vi "SnapShoot.vi"(8 "error in (no error)":errorcluster, 11 "CameraTestingProxy in":refnum<class "CameraTestingProxyAPI.lvclass">) -> (0 "error out":errorcluster, 2 "SnapData":T1, 3 "CameraTestingProxy out":refnum<class "CameraTestingProxyAPI.lvclass">)   [LabVIEW 2020, in "CameraTestingProxy.lvlib" / "CameraTestingProxyAPI.lvclass"]
uses:
  CameraTestingProxyAPI.lvclass
  ICameraTestingProxy/TypeDef/SnapData.ctl
  ICameraTestingProxy/TypeDef/Resolution.ctl
  CameraTestingProxyAPI.lvclass/CameraTestingProxyAPI.ctl
  81c5d912-67c1-434d-ab51-26c85ecb9ac1.vi
  ICameraTestingProxy/TypeDef/ICameraTestingProxy_typedef.lvlib
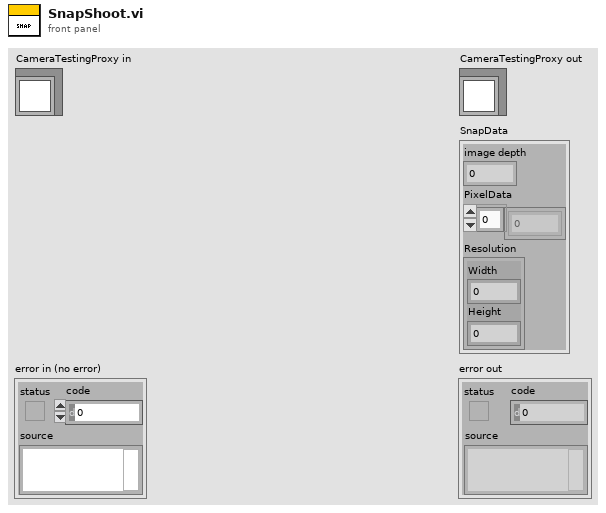
[diagram p1: front panel]
types:
  T1 = typedef "ICameraTestingProxy_typedef.lvlib/SnapData.ctl" = cluster{"image depth":i32, "PixelData":u8[], "Resolution":T2}
  T2 = typedef "ICameraTestingProxy_typedef.lvlib/Resolution.ctl" = cluster{"Width":i16, "Height":i16}
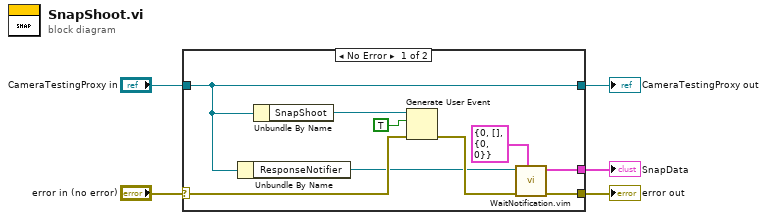
[diagram p0: block diagram]
diagram:
  n1 = case shown="No Error" "error in (no error)" {
    selector: "error in (no error)" -> [w13 w16]
    tunnel: [w9 w16] -> w2
    tunnel: [w8 w15] -> w4
    tunnel: "CameraTestingProxy in" -> [w8 w15]
    tunnel: [w10 _] -> w3
    frame No Error {
      n2 = Unbundle By Name(w8) -> ("ResponseNotifier"=w7:refnum<notifier>)
      n3 = Unbundle By Name(w8) -> ("SnapShoot"=w14:refnum<user-event>)
      n4 = Generate User Event(user event=w14, event data cluster=TRUE ("event data"), error in=w13) -> (error out=w11:errorcluster)  [unwired: 1 in, 1 out]
      n5 = call "WaitNotification.vim"("Type"=T1 {"image depth"=0, "PixelData"=[], "Resolution"={"Width"=0, "Height"=0}} ("SnapData"), "error in (no error)"=w11, "ResponseNotifier"=w7) -> ("error out"=w9:errorcluster, "Data"=w10:T1)  [unwired: 6 in, 1 out]
    }
    frame Error {
    }
  }
  "error out" <- w2
  "CameraTestingProxy out" <- w4
  "SnapData" <- w3
